vi "DB - [Config].[Messages].vi"(0 "connection reference":T2, 1 "DB Connection":T3={"Open"=TRUE, "Close"=TRUE}, 2 "INSERT TO [SRTRS].[Execute].[MessageLog]":bool, 3 "Application (Default SRTRS)":string="SRTRS", 5 "INSERT TO [AMS].[Execute].[MessageLog]":bool, 7 "Cluster (When DB Not Available)":T1, 9 "<.?...> + Pre-Description<PrePost>Post-Description":string, 11 "error in (no error)":errorcluster) -> (4 "connection reference":T2, 6 "OK Out":bool caption="OK1", 8 "<NoD>":bool, 12 "[Remarks] Pre+Description+Post (Unicode)":string, 13 "Message Code <. ....> FOUND":bool, 14 "[ShortDescription] (Unicode)":string, 15 "SUMMARY":errorcluster)   [LabVIEW 2013]
uses:
  <vilib>/addons/database/Connection.llb/Conn ObjectReference.ctl
  Controls/DB - OpenClose.ctl
  Controls/DB - [SRTRS].[Execute].[MessageLog] ColNames.ctl
  Controls/DB - [AMS].[Execute].[Message] ColNames.ctl
  Controls/Global SRTRS.vi
  <vilib>/addons/database/Connection.llb/DB Tools Open Connec (String).vi
  Controls/Global CMS.vi
  Controls/Global AMS.vi
  <vilib>/addons/database/Connection.llb/Conn Execute.vi
  <vilib>/addons/database/Recordset.llb/Rec Destroy - Connection.vi
  <vilib>/addons/database/NI_Database_API.lvlib
panel:
  out "Config.SG,UG,UGR,Users":string[][](array[string])
  out "Config.SG,UG,UGR,Users":errorcluster
  out "GetNewMessageLogNo":errorcluster
  out "AMS.Execute.Message":errorcluster
  out "[SRTRS].[Execute].[MessageLogNo]":string
  out "AMS.Execute.Message":string="AMS.Execute.MessageLog"
  out "SQL Statement":string[](array[string])
  out "<NoML>":bool
  out "<.....>+ Pre+Description+Post (Unicode)":string
  out "[ShortDescription]":string
  out "[SeverityLevel]":string
  out "Execute.MessageLog":errorcluster
  out "Config.Messages":errorcluster
  out "[MessageId]":string
  out "[MessageType]":string
  out "DB Close Error":errorcluster
  out "Config.Messages":string[](array[string])
  out "DB.Execute.MessageLog":string="SRTRS.Execute.MessageLog"
  out "DB.Config.Messages":string="SRTRS.Config.Messages"
  out "Connection Information":T4={"Connection "="SQL Server 32bit HPEnvy", "Username"="admin", "Password"="admin123"}
  # "<E 602> Hold Temperature Exceeded Variant Allowed!"
  # "Test Codes\nComments\nNeed to set \nPlant, Language\nEnable INSERTS when testing"
  # "<I0101>Admin\n<E7105> Operator<PrePost>4070\n<E8107> Database Not Not Available  (en and zh)"
  # "3C45 2032 3033 3EA2 5B37 620D 54F0 79"
  # "<E7203>ÿþÿþ¢[7b\nTðy Å_{eQ0"
  # "<E 203>¢[7b\nTðy"
  # "[SeverityLevel]                                   [ShortDescription]"
  # "sg.[SeverityGroupId]  ,ug.[UserGroupId] ,ug.[SendSms]  ,ug.[SendEmail]   ,ugr.[UserId]      ,u.[MobileNo]          ,u.[Email]"
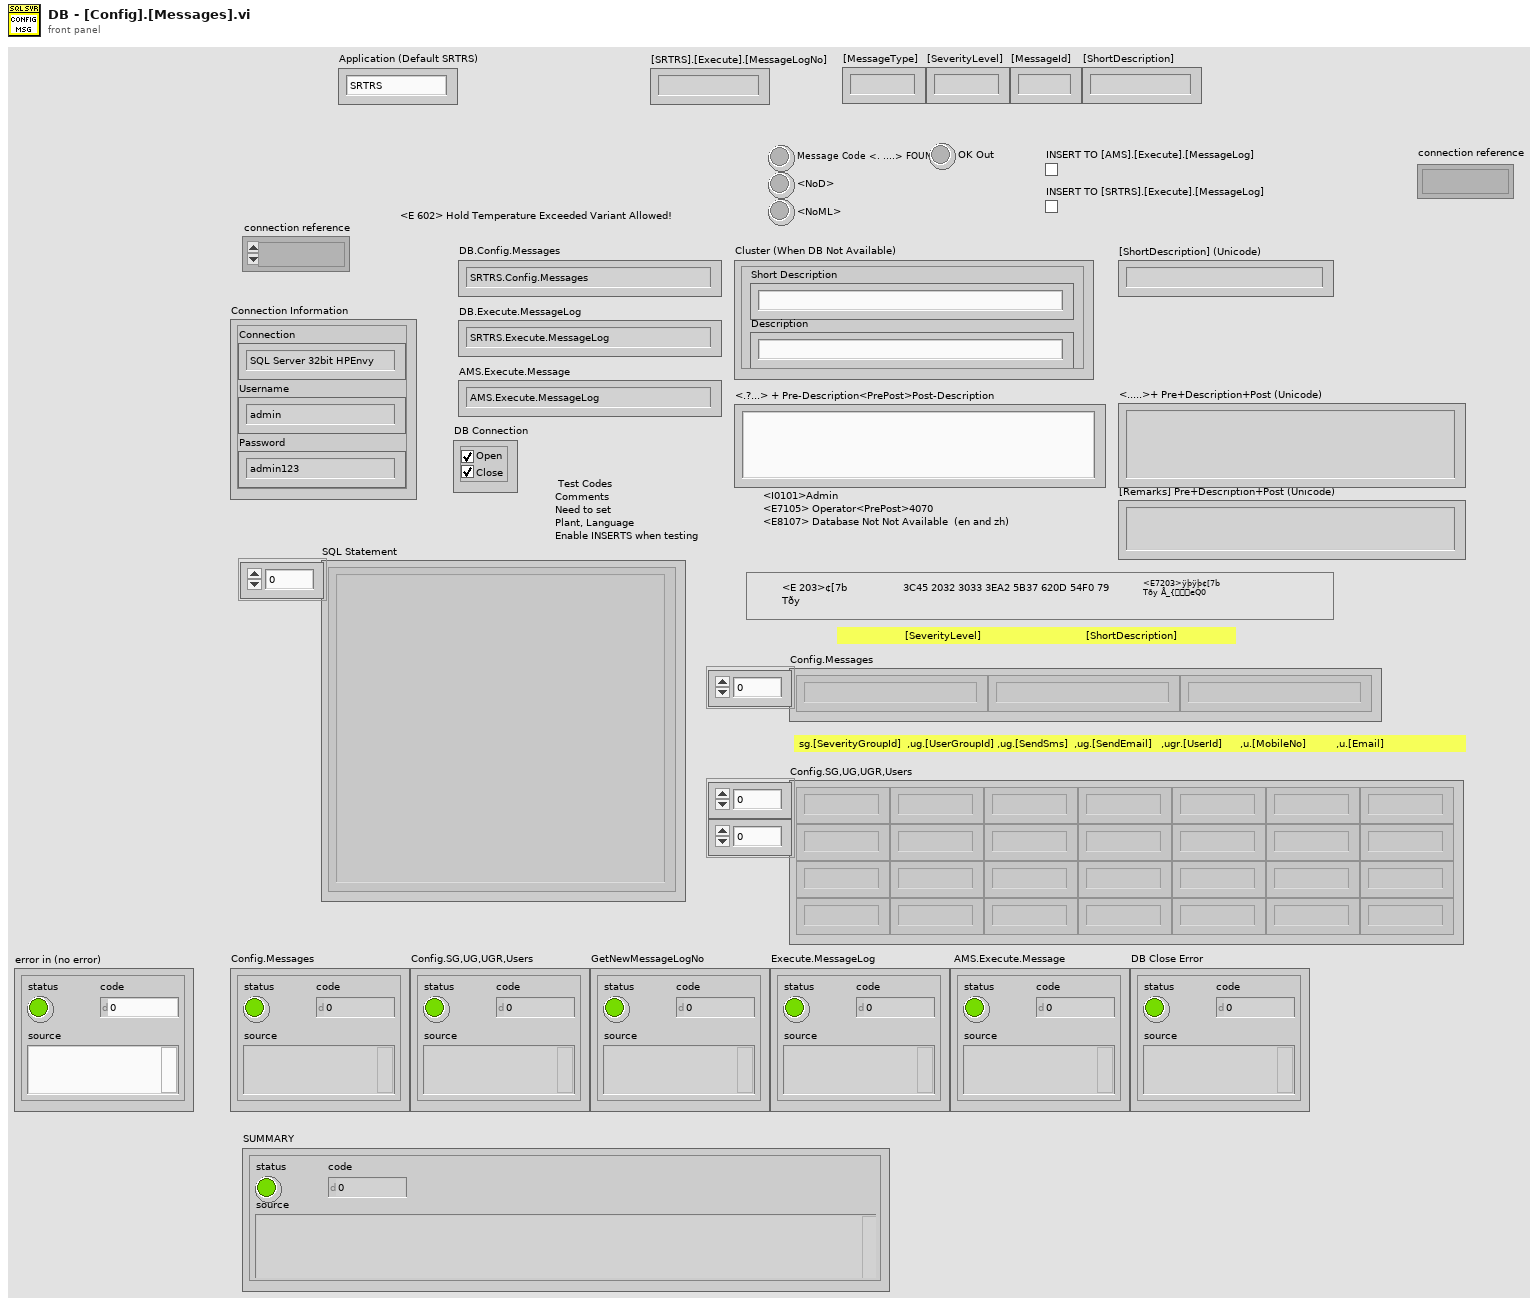
[diagram p1: front panel]
types:
  T1 = cluster{"Short Description":string, "Description":string}
  T2 = typedef "NI_Database_API.lvlib/Conn ObjectReference.ctl" = refnum<k1>
  T3 = typedef "DB - OpenClose.ctl" = cluster{"Open":bool, "Close":bool}
  T4 = cluster{"Connection ":string, "Username":string, "Password":string}
  T5 = typedef "Enum - InteractiveMode-SubVIMode.ctl" = enum16{"Interactive", "subVI Mode"}
  T6 = typedef "DB - Logon Extra Info.ctl" = cluster{"Plant Name":string, "UserName":string, "Hostname [ClientName]":string, "IsUnicode":bool}
  T7 = typedef "Connection Information Cluster.ctl" = cluster{"Connection ":string, "Username":string, "Password":string}
  T8 = typedef "DB - [AMS].[Execute].[Message] ColNames.ctl" = enum16{"[MessageNo]", "[LanguageId]", "[SoftwareSolutionId]", "[SoftwareSolutionName]", "[PlantId]", "[SystemId]", "[StationId]", "[MessageLogNo]", "[ReceivedOn]", "[MessageCode]", "[ShortDescription]", "[Message]", "[SmsMessage]", "[SuppMessage1]", "[SuppMessage2]", "[SuppMessage3]", "[TransactionNo]", "[TransactionRunNo]", "[MessageInitiator]", "[Remarks]", "[MsgCreatedOn]", "[IsToSendSms]", "[IsToSendEmail]", "[IsToSendCommMedium1]", "[IsToSendCommMedium2]", "[SmsContent]", "[EmailContent]", "[CommMed1Content]", "[CommMed2Content]", "[MobileNos]", "[EmailAddresses]", "[CommMedium1Ids]", "[CommMedium2Ids]", "[LastAttemptedCommMed]", "[LastAttemptedNo]", "[LastAttemptedOn]", "[IsSmsSent]", "[IsEmailSent]", "[IsCommMedium1Sent]", "[IsCommMedium2Sent]", "[OverallSentStatus]", "[StatusUpdatedOn]", "[IsArchived]"}
  T9 = typedef "DB - [SRTRS].[Execute].[MessageLog] ColNames.ctl" = enum16{"[MessageLogNo]", "[MessageType]", "[MessageId]", "[SeverityLevel]", "[PlantId]", "[StationId]", "[UserId]", "[TransactionNo]", "[TransactionRunNo]", "[Message]", "[Remarks]", "[CreatedOn]", "[SendRequired]", "[SentOn]", "[OverallMsgStatus]", "[StatusUpdatedOn]", "[IsArchived]"}
  T10 = typedef "DB - Logon Info.ctl" = cluster{"PlantID":string, "SystemID":string, "UserID":string, "DomainID":string, "LanguageID":string, "StationID":string}
  T11 = typedef "DB - DB.Schema.Table.ctl" = cluster{"DB":string, "Schema":string, "Table":string}
  T12 = typedef "NI_Database_API.lvlib/Rec ObjectReference.ctl" = refnum<k1>
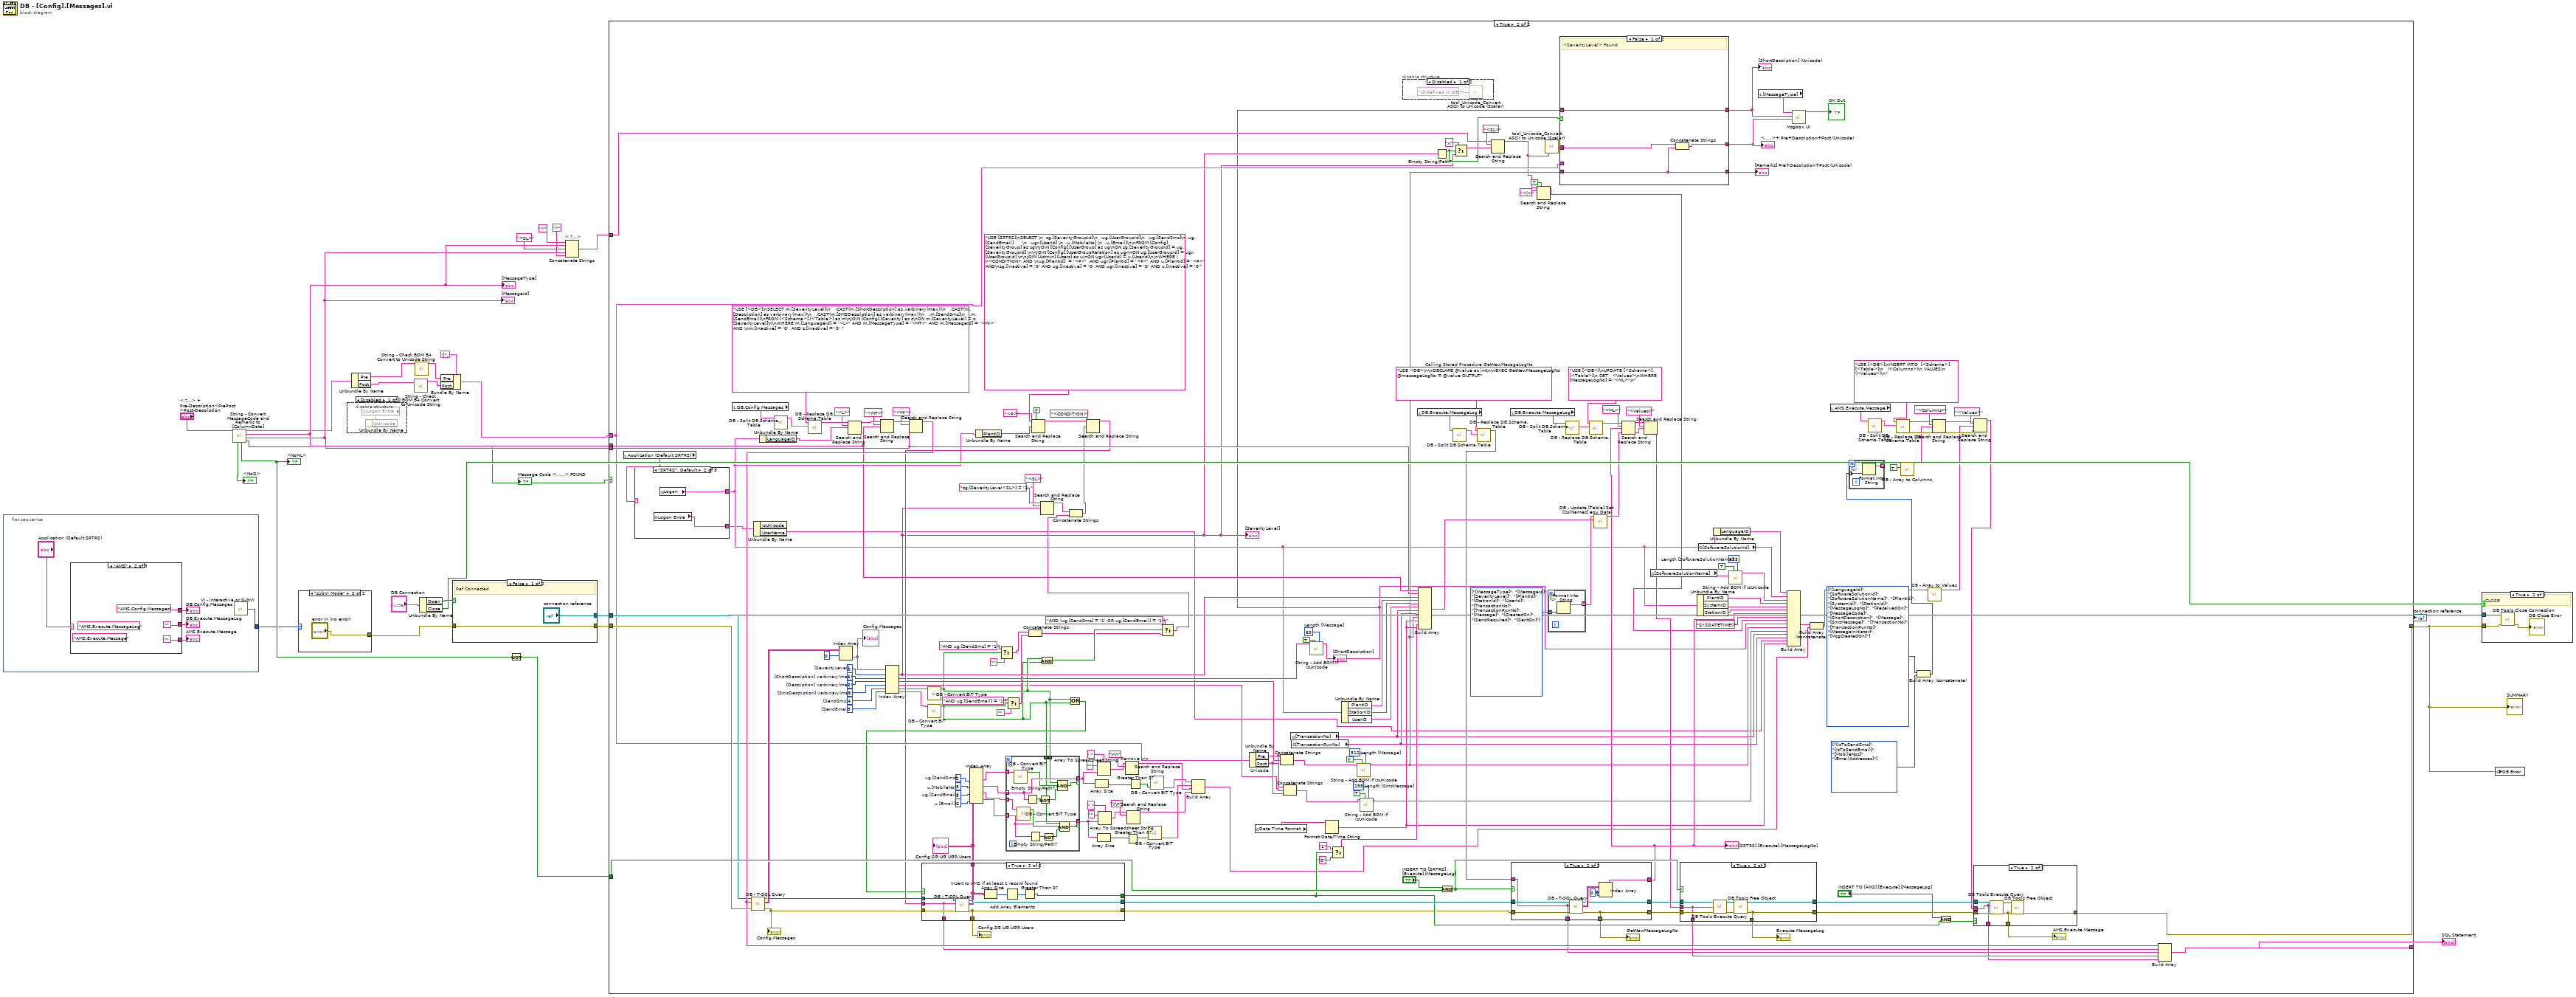
[diagram p0: block diagram]
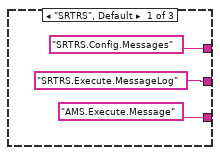
[diagram p2: hidden frame]
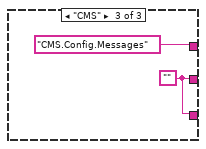
[diagram p3: hidden frame]
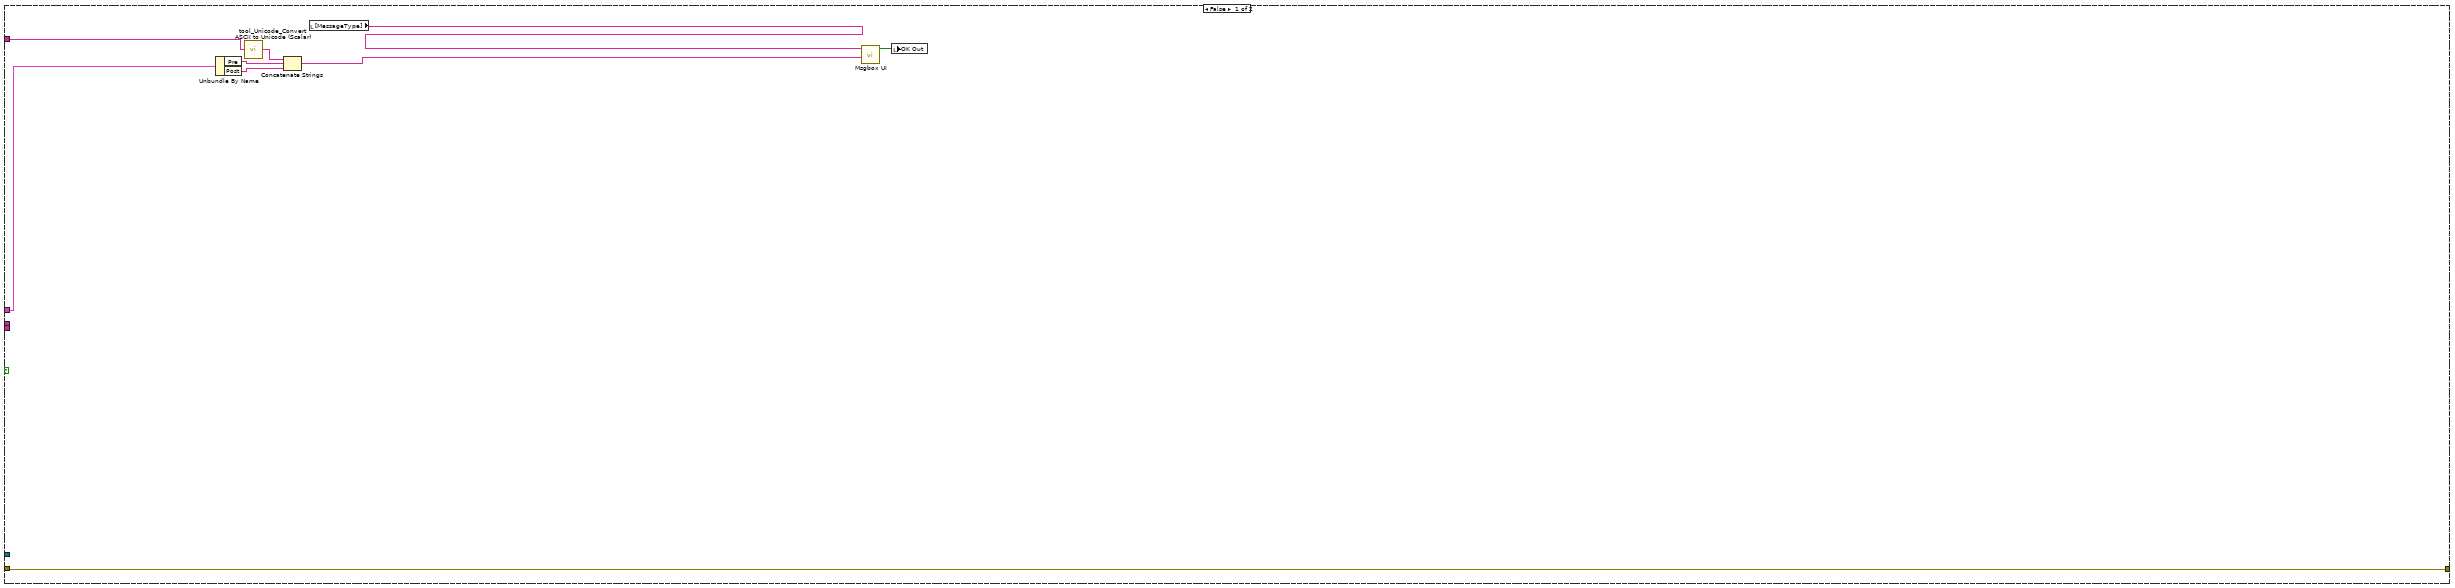
[diagram p5: hidden frame]
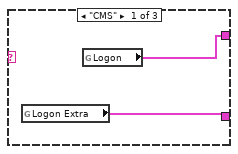
[diagram p6: hidden frame]
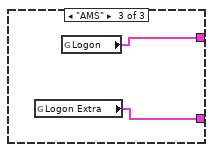
[diagram p7: hidden frame]
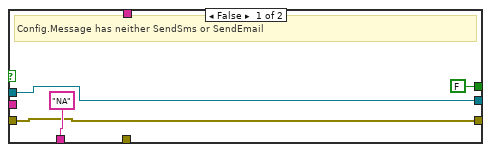
[diagram p8: hidden frame]
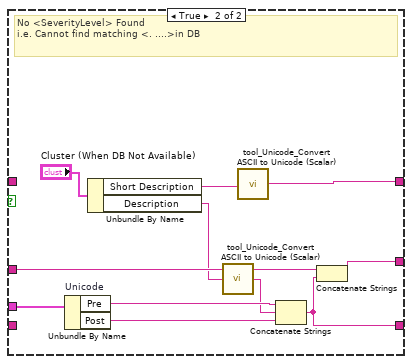
[diagram p9: hidden frame]
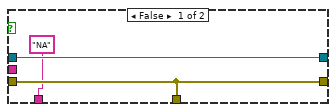
[diagram p11: hidden frame]
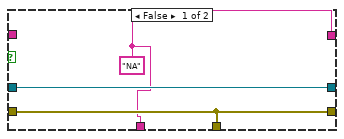
[diagram p12: hidden frame]
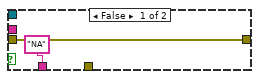
[diagram p13: hidden frame]
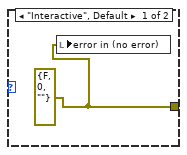
[diagram p15: hidden frame]
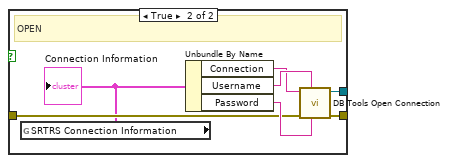
[diagram p16: hidden frame]
diagram:
  n1 = flat-sequence {
    tunnel: [w28] -> w1
    frame #0 {
      n2 = case shown="\"AMS\"" "Application (Default SRTRS)" {
        tunnel: ["SRTRS.Config.Messages" ("SRTRS.Config.Messages") "AMS.Config.Messages" ("SRTRS.Config.Messages") "CMS.Config.Messages" ("SRTRS.Config.Messages")] -> w31
        tunnel: ["SRTRS.Execute.MessageLog" ("SRTRS.Execute.MessageLog") "" w39] -> w30
        tunnel: ["AMS.Execute.Message" ("AMS.Execute.MessageLog") "" w39] -> w29
        frame "SRTRS", Default {
        }
        frame "AMS" {
          (unwired) "AMS.Execute.Message" ("SRTRS.Config.Messages")
          (unwired) "AMS.Execute.MessageLog" ("SRTRS.Config.Messages")
        }
        frame "CMS" {
          w39 = ""
        }
      }
      "DB.Config.Messages" <- w31
      "DB.Execute.MessageLog" <- w30
      "AMS.Execute.Message" <- w29
      n3 = call "VI - Interactive or SubVI.vi"() -> ("Mode"=w28:T5)  [unwired: 5 in]
    }
  }
  n4 = call "String - Convert MessageCode and Remarks to [ColumnData].vi"("<. ....> + Pre-Description<PrePost>Post-Description"="<.?...> + Pre-Description<PrePost>Post-Description") -> ("Message Code <.....> Found"=w10:bool, "[MessageId]"=w18:string, "[MessageType]"=w19:string, "PrePost Description"=w4:cluster{"Pre":string, "Post":string}, "<NoML>"=w11:bool, "<NoD>"=→"<NoD>":bool)  [unwired: 4 in, 1 out]
  "[MessageType]" <- w19
  "[MessageId]" <- w18
  "Message Code <. ....> FOUND" <- w10
  "<NoML>" <- w11
  n5 = case shown="\"subVI Mode\"" w1 {
    tunnel: [w41 "error in (no error)"] -> w25
    frame "Interactive", Default {
      w41 = errorcluster {"status"=FALSE, "code"=0, "source"=""} ("error in (no error)")
      n6 = local write "error in (no error)"(w41) -> ()
    }
    frame "subVI Mode" {
    }
  }
  n7 = disable-structure shown="Disabled" {
    frame Disabled {
      n8 = global read "Global SRTRS.vi" "Logon Extra"() -> (w43:T6)
      n9 = Unbundle By Name(w43) -> ()  [unwired: 1 out]
    }
    frame Enabled {
    }
  }
  n10 = Unbundle By Name ("Depends on IsUnicode")(w4) -> ("Pre"=w7:string, "Post"=w8:string)
  n11 = call "String - Check BOM B4 Convert to Unicode String.vi"("Check 0xFFEE"=w8) -> ("Convert ASCII to Unicode"=w5:string)  [unwired: 10 in]
  n12 = call "String - Check BOM B4 Convert to Unicode String.vi"("Check 0xFFEE"=w7) -> ("Convert ASCII to Unicode"=w6:string)  [unwired: 10 in]
  n13 = Unbundle By Name("DB Connection") -> ("Open"=w26:bool, "Close"=w23:bool)
  n14 = Bundle By Name(cluster=cluster{"Pre":string, "Post":string} {"Pre"="", "Post"=""} ("input cluster"), "Pre"=w6, "Post"=w5) -> (w2:cluster{"Pre":string, "Post":string})
  n15 = case shown="False" w26 {
    tunnel: ["connection reference" w49] -> w12
    tunnel: w25 -> [w44 w48]
    tunnel: [w44 w47] -> w24
    frame False {
      # "Ref Connected"
    }
    frame True {
      # "OPEN"
      n16 = global read "Global SRTRS.vi" "SRTRS Connection Information"() -> (w46:T7)
      "Connection Information" <- w46
      n17 = Unbundle By Name(w46) -> ("Connection"=w51:string, "Username"=w52:string, "Password"=w50:string)
      n18 = call-poly <vilib>:"DB Tools Open Connection.vi"("password"=w50, "userID"=w52, "error in (no error)"=w48, "connection information"=w51) -> ("error out"=w47:errorcluster, "connection reference"=w49:T2)  [unwired: 4 in]
    }
  }
  "connection reference" <- w12
  n19 = Not(x=w11) -> (.not. x?=w15:bool)
  n20 = Concatenate Strings "<.?...>"("<" ("string"), w19, "<SL>" ("search string"), w18, ">" ("string")) -> (w9:string)
  n21 = case shown="True" w10 {
    tunnel: w24 -> [w61 w255]
    tunnel: [w61 w215] -> w21
    tunnel: w19 -> [_ w204]
    tunnel: w18 -> [_ w203]
    tunnel: w15 -> [_ w244]
    tunnel: [_ w243] -> w13
    tunnel: w12 -> [_ w242]
    tunnel: w2 -> [w59 w178]
    tunnel: w9 -> [w55 w185]
    frame False {
      n22 = Unbundle By Name(w59) -> ("Pre"=w58:string, "Post"=w57:string)
      n23 = call "tool_Unicode_Convert ASCII to Unicode (Scalar).vi"("ASCII"=w55) -> ("Unicode"=w54:string)  [unwired: 4 in]
      n24 = Concatenate Strings(w54, w58, w57) -> (w53:string)
      n25 = local read "[MessageType]"() -> (w60:string)
      n26 = call "Msgbox UI.vi"("<xxxxxx> + Pre+Description+Post (Unicode)"=w53, "[MessageType]"=w60) -> ("OK Out"=w56:bool)  [unwired: 7 in, 2 out]
      n27 = local write "OK Out"(w56) -> ()
    }
    frame True {
      w85 = 60  # Length [Message]
      w91 = 255  # Length [SoftwareSolutionName]
      w111 = 5  # [SendEmail
      w112 = 4  # [SendSms]
      w135 = 3  # ug.[SendEmail]
      w139 = 2  # ug.[SendSms]
      w147 = T8[] [enum."[IsToSendSms]", enum."[IsToSendEmail]", enum."[MobileNos]", enum."[EmailAddresses]"] items=["[MessageNo]", "[LanguageId]", "[SoftwareSolutionId]", "[SoftwareSolutionName]", "[PlantId]", "[SystemId]", "[StationId]", "[MessageLogNo]", "[ReceivedOn]", "[MessageCode]", "[ShortDescription]", "[Message]", "[SmsMessage]", "[SuppMessage1]", "[SuppMessage2]", "[SuppMessage3]", "[TransactionNo]", "[TransactionRunNo]", "[MessageInitiator]", "[Remarks]", "[MsgCreatedOn]", "[IsToSendSms]", "[IsToSendEmail]", "[IsToSendCommMedium1]", "[IsToSendCommMedium2]", "[SmsContent]", "[EmailContent]", "[CommMed1Content]", "[CommMed2Content]", "[MobileNos]", "[EmailAddresses]", "[CommMedium1Ids]", "[CommMedium2Ids]", "[LastAttemptedCommMed]", "[LastAttemptedNo]", "[LastAttemptedOn]", "[IsSmsSent]", "[IsEmailSent]", "[IsCommMedium1Sent]", "[IsCommMedium2Sent]", "[OverallSentStatus]", "[StatusUpdatedOn]", "[IsArchived]"]
      w87 = 255  # Length [SmsMessage]
      w149 = 3  # [SmsDescription] varbinary(max)
      w134 = 6  # u.[Email]
      w137 = 5  # u.[MobileNo]
      w192 = 2  # [Description] varbinary(max)
      w88 = 512  # Length [Message]
      w145 = T8[] [enum."[LanguageId]", enum."[SoftwareSolutionId]", enum."[SoftwareSolutionName]", enum."[PlantId]", enum."[SystemId]", enum."[StationId]", enum."[MessageLogNo]", enum."[ReceivedOn]", enum."[MessageCode]", enum."[ShortDescription]", enum."[Message]", enum."[SmsMessage]", enum."[TransactionNo]", enum."[TransactionRunNo]", enum."[MessageInitiator]", enum."[MsgCreatedOn]"] items=["[MessageNo]", "[LanguageId]", "[SoftwareSolutionId]", "[SoftwareSolutionName]", "[PlantId]", "[SystemId]", "[StationId]", "[MessageLogNo]", "[ReceivedOn]", "[MessageCode]", "[ShortDescription]", "[Message]", "[SmsMessage]", "[SuppMessage1]", "[SuppMessage2]", "[SuppMessage3]", "[TransactionNo]", "[TransactionRunNo]", "[MessageInitiator]", "[Remarks]", "[MsgCreatedOn]", "[IsToSendSms]", "[IsToSendEmail]", "[IsToSendCommMedium1]", "[IsToSendCommMedium2]", "[SmsContent]", "[EmailContent]", "[CommMed1Content]", "[CommMed2Content]", "[MobileNos]", "[EmailAddresses]", "[CommMedium1Ids]", "[CommMedium2Ids]", "[LastAttemptedCommMed]", "[LastAttemptedNo]", "[LastAttemptedOn]", "[IsSmsSent]", "[IsEmailSent]", "[IsCommMedium1Sent]", "[IsCommMedium2Sent]", "[OverallSentStatus]", "[StatusUpdatedOn]", "[IsArchived]"]
      w225 = "USE <DB>\n\nDECLARE @value as int\n\nEXEC GetNewMessageLogNo  @messageLogNo = @value OUTPUT"  # Calling Stored Procedure GetNewMesageLogNo
      w229 = T9[] [enum."[MessageType]", enum."[MessageId]", enum."[SeverityLevel]", enum."[PlantId]", enum."[StationId]", enum."[UserId]", enum."[TransactionNo]", enum."[TransactionRunNo]", enum."[Message]", enum."[CreatedOn]", enum."[SendRequired]", enum."[SentOn]"] items=["[MessageLogNo]", "[MessageType]", "[MessageId]", "[SeverityLevel]", "[PlantId]", "[StationId]", "[UserId]", "[TransactionNo]", "[TransactionRunNo]", "[Message]", "[Remarks]", "[CreatedOn]", "[SendRequired]", "[SentOn]", "[OverallMsgStatus]", "[StatusUpdatedOn]", "[IsArchived]"]
      w235 = 1  # [ShortDescription] varbinary(max)
      w239 = 0  # [SeverityLevel]
      n28 = local read "Application (Default SRTRS)"() -> (w80:string)
      n29 = case shown="\"SRTRS\", Default" w80 {
        tunnel: [w257 w259 w261] -> w79
        tunnel: [w256 w258 w260] -> w72
        frame "CMS" {
          n30 = global read "Global CMS.vi" "Logon Extra"() -> (w256:T6)
          n31 = global read "Global CMS.vi" "Logon"() -> (w257:T10)
        }
        frame "SRTRS", Default {
          n32 = global read "Global SRTRS.vi" "Logon Extra"() -> (w258:T6)
          n33 = global read "Global SRTRS.vi" "Logon"() -> (w259:T10)
        }
        frame "AMS" {
          n34 = global read "Global AMS.vi" "Logon Extra"() -> (w260:T6)
          n35 = global read "Global AMS.vi" "Logon"() -> (w261:T10)
        }
      }
      n36 = local read "DB.Config.Messages"() -> (w177:string)
      n37 = Unbundle By Name(w72) -> ("UserName"=w67:string)  [unwired: 1 out]
      n38 = Unbundle By Name(w79) -> ("LanguageID"=w233:string)
      n39 = call "DB - Split DB.Schema.Table.vi"("DB.Schema.Table"=w177) -> ("DB.Schema.Table"=w254:T11)  [unwired: 10 in]
      n40 = call "DB - Replace DB.Schema.Table.vi"("DB.Schema.Table"=w254, "string in"="USE [<DB>]\nSELECT m.[SeverityLevel]\n   ,CAST(m.[ShortDescription] as varbinary(max))\n   ,CAST(m.[Description] as varbinary(max))\n   ,CAST(m.[SMSDescription] as varbinary(max))\n   ,m.[SendSms]\n   ,m.[SendEmail]\nFROM [<Schema>].[<Table>] as m\nJOIN [Config].[Severity] as c\nON m.[SeverityLevel] = c.[SeverityLevel]\n\nWHERE m.[LanguageId] = '<L>' AND m.[MessageType] = '<MT>' AND m.[MessageId] = '<MI>' AND \nm.[Inactive] = '0'  AND c.[Inactive] = '0' ") -> ("string out"=w252:string)  [unwired: 8 in, 1 out]
      n41 = Search and Replace String(input string=w252, search string="<L>", replace string=w233) -> (result string=w250:string)  [unwired: 5 in, 3 out]
      n42 = Search and Replace String(input string=w250, search string="<MT>", replace string=w204) -> (result string=w248:string)  [unwired: 5 in, 3 out]
      n43 = Search and Replace String(input string=w248, search string="<MI>", replace string=w203) -> (result string=w247:string)  [unwired: 5 in, 3 out]
      n44 = call "DB - T-SQL Query.vi"("error in (no error)"=w255, "T-SQL"=w247, "connection reference"=w242) -> ("error out"=w170:errorcluster, "2D data"=w234:string[][], "connection reference"=w171:T2)  [unwired: 6 in]
      "Config.Messages" <- w170
      n45 = Index Array(array=w234, index (row)=0) -> (element=w240:string[])  [unwired: 1 in]
      "Config.Messages" <- w240
      n46 = Index Array(array=w240, index #1=w239, index #2=w235, index #3=w192, index #4=w149, index #5=w112, index #6=w111) -> (element #1=w113:string, element #2=w84:string, element #3=w191:string, element #4=w63:string, element #5=w110:string, element #6=w109:string)
      "[SeverityLevel]" <- w113
      n47 = call "DB - Convert BIT Type.vi"("BIT Type (eg Inactive)"=w110) -> ("Boolean"=w74:bool)  [unwired: 2 in, 2 out]
      n48 = call "DB - Convert BIT Type.vi"("BIT Type (eg Inactive)"=w109) -> ("Boolean"=w73:bool)  [unwired: 2 in, 2 out]
      n49 = Unbundle By Name(w79) -> ("PlantID"=w172:string)
      n50 = Select(t="AND ug.[SendSms] = '1'" ("string (\"\")"), s=w74, f="") -> (s? t:f=w103:string)
      n51 = Select(t="AND ug.[SendEmail] = '1'" ("string (\"\")"), s=w73, f="") -> (s? t:f=w102:string)
      n52 = Concatenate Strings(w103, w102) -> (w76:string)
      n53 = Search and Replace String(replace all?=TRUE ("replace all? (F)"), input string="USE [SRTRS]\nSELECT \n  sg.[SeverityGroupId]\n  ,ug.[UserGroupId]\n  ,ug.[SendSms]\n ,ug.[SendEmail]      \n  ,ugr.[UserId] \n  ,u.[MobileNo] \n  ,u.[Email]\n\nFROM [Config].[SeverityGroup] as sg\nJOIN [Config].[UserGroup] as ug\nON sg.[SeverityGroupId] = ug.[SeverityGroupId] \n\nJOIN [Config].[UserGroupRelation] as ugr\nON ug.[UserGroupId] = ugr.[UserGroupId] \n\nJOIN [Admin].[Users] as u\nON ugr.[UserId] = u.[UserId]\n\nWHERE \n<CONDITION> AND \nug.[PlantId]  = '<P>'  AND ugr.[PlantId] = '<P>' AND u.[PlantId] = '<P>' AND\nsg.[Inactive] = '0' AND ug.[Inactive] = '0' AND ugr.[Inactive] = '0' AND u.[Inactive] = '0'", search string="<P>", replace string=w172) -> (result string=w141:string)  [unwired: 4 in, 3 out]
      n54 = Search and Replace String(input string="sg.[SeverityLevel<SL>] = '1' " ("search string"), search string="<SL>" ("replace string (\"\")"), replace string=w113) -> (result string=w104:string)  [unwired: 5 in, 3 out]
      n55 = And(x=w74, y=w73) -> (x .and. y?=w78:bool)
      n56 = Or(x=w74, y=w73) -> (x .or. y?=w98:bool)
      n57 = Select(t="AND (ug.[SendSms] = '1' OR ug.[SendEmail] = '1') " ("string (\"\")"), s=w78, f=w76) -> (s? t:f=w75:string)
      n58 = Concatenate Strings(w104, w75) -> (w101:string)
      n59 = Search and Replace String(input string=w141, search string="<CONDITION>", replace string=w101) -> (result string=w120:string)  [unwired: 5 in, 3 out]
      n60 = case shown="True" w98 {
        tunnel: w171 -> [w262 w274]
        tunnel: w170 -> [w264 w273]
        tunnel: [_ w266] -> w169
        tunnel: [w262 w272] -> w168
        tunnel: [FALSE w269] -> w167
        tunnel: [_ w268] -> w163
        tunnel: w120 -> [_ w267]
        tunnel: ["NA" ("result string") w267] -> w100
        tunnel: [w264 w266] -> w99
        frame False {
          # "Config.Message has neither SendSms or SendEmail"
        }
        frame True {
          n61 = call "DB - T-SQL Query.vi"("error in (no error)"=w273, "T-SQL"=w267, "connection reference"=w274) -> ("error out"=w266:errorcluster, "2D data"=w268:string[][], "connection reference"=w272:T2)  [unwired: 6 in]
          n62 = Array Size "Insert to AMS if at least 1 record found"(array=w268) -> (size(s)=w271:i32[])
          n63 = Add Array Elements(numeric array=w271) -> (sum=w270:i32)
          n64 = Greater Than 0?(x=w270) -> (x > 0?=w269:bool)
        }
      }
      "Config.SG,UG,UGR,Users" <- w169
      "Config.SG,UG,UGR,Users" <- w163
      n65 = Index Array(array=w163, index (col) #1=w139, index (col) #2=w137, index (col) #3=w135, index (col) #4=w134) -> (element #1=w138:string[], element #2=w136:string[], element #3=w133:string[], element #4=w132:string[])  [unwired: 4 in]
      n66 = for {
        tunnel: w138 -> [w288] mode=indexing
        tunnel: w136 -> [w287] mode=indexing
        tunnel: [w287] -> w131 mode=indexing if=w283
        tunnel: w133 -> [w282] mode=indexing
        tunnel: w132 -> [w278] mode=indexing
        tunnel: [w278] -> w130 mode=indexing if=w277
        tunnel: w74 -> [w276]
        tunnel: w73 -> [w275]
        n67 = call "DB - Convert BIT Type.vi"("BIT Type (eg Inactive)"=w288) -> ("Boolean"=w285:bool)  [unwired: 2 in, 2 out]
        n68 = call "DB - Convert BIT Type.vi"("BIT Type (eg Inactive)"=w282) -> ("Boolean"=w280:bool)  [unwired: 2 in, 2 out]
        n69 = Empty String/Path?(string/path=w287) -> (empty?=w286:bool)
        n70 = Empty String/Path?(string/path=w278) -> (empty?=w281:bool)
        n71 = Not(x=w286) -> (.not. x?=w284:bool)
        n72 = Not(x=w281) -> (.not. x?=w279:bool)
        n73 = Compound Arithmetic op=AND(w276, w285, w284) -> (w283:bool)
        n74 = Compound Arithmetic op=AND(w275, w280, w279) -> (w277:bool)
      }
      n75 = Array Size(array=w131) -> (size(s)=w129:i32)
      n76 = Array To Spreadsheet String(delimiter (Tab)=",", array=w131, 3:"" ("format string")) -> (spreadsheet string=w156:string)
      n77 = Array Size(array=w130) -> (size(s)=w128:i32)
      n78 = Array To Spreadsheet String(delimiter (Tab)=",", array=w130, 3:"" ("format string")) -> (spreadsheet string=w157:string)
      n79 = Search and Replace String "Remove \\r\\n"(input string=w156, search string="\r\n") -> (result string=w123:string)  [unwired: 6 in, 3 out]
      n80 = Greater Than 0?(x=w128) -> (x > 0?=w126:bool)
      n81 = Search and Replace String(input string=w157, search string="\r\n") -> (result string=w122:string)  [unwired: 6 in, 3 out]
      n82 = Greater Than 0?(x=w129) -> (x > 0?=w127:bool)
      n83 = call "DB - Convert BIT Type.vi"("Boolean"=w126) -> ("BIT (eg Inactive)"=w124:string)  [unwired: 2 in, 2 out]
      n84 = call "DB - Convert BIT Type.vi"("Boolean"=w127) -> ("BIT (eg Inactive)"=w125:string)  [unwired: 2 in, 2 out]
      n85 = Build Array(w125, w124, w123, w122) -> (w121:string[])
      n86 = Unbundle By Name "Unicode"(w178) -> ("Pre"=w65:string, "Post"=w64:string)
      n87 = global read "Global SRTRS.vi" "Date Time Format"() -> (w237:string)
      n88 = Concatenate Strings(w65, w191, w64) -> (w90:string)
      n89 = Concatenate Strings(w65, w63, w64) -> (w62:string)
      n90 = global read "Global SRTRS.vi" "[TransactionNo]"() -> (w197:string)
      n91 = global read "Global SRTRS.vi" "[TransactionRunNo]"() -> (w196:string)
      n92 = call "String - Add BOM if IsUnicode.vi"("target length (65535)"=w85, "Input is Unicode (varbinary)?"=TRUE ("IsUnicode?"), "String IN"=w84) -> ("BOM Added"=w83:string)  [unwired: 8 in]
      "[ShortDescription]" <- w83
      n93 = Format Date/Time String(time format string (%c)=w237) -> (date/time string=w148:string)  [unwired: 2 in]
      n94 = Select(t="1", s=w167, f="0") -> (s? t:f=w164:string)
      n95 = Unbundle By Name(w79) -> ("PlantID"=w202:string, "StationID"=w198:string, "UserID"=w66:string)
      n96 = call "String - Add BOM if IsUnicode.vi"("target length (65535)"=w88, "Input is Unicode (varbinary)?"=TRUE, "String IN"=w90) -> ("BOM Added"=w89:string)  [unwired: 8 in]
      n97 = call "String - Add BOM if IsUnicode.vi"("target length (65535)"=w87, "Input is Unicode (varbinary)?"=TRUE, "String IN"=w62) -> ("BOM Added"=w86:string)  [unwired: 8 in]
      n98 = disable-structure shown="Disabled" {
        frame Disabled {
          n99 = call "tool_Unicode_Convert ASCII to Unicode (Scalar).vi"("ASCII"="Undefined in DB.") -> ()  [unwired: 4 in, 1 out]
        }
        frame Enabled {
        }
      }
      n100 = local read "DB.Execute.MessageLog"() -> (w176:string)
      n101 = Build Array(w204, w203, w113, w202, w198, w66, w197, w196, w89, w148, w164, w148) -> (w230:string[])
      n102 = Empty String/Path?(string/path=w113) -> (empty?=w181:bool)
      n103 = And(x="INSERT TO [SRTRS].[Execute].[MessageLog]", y=w244) -> (x .and. y?=w194:bool)
      n104 = call "DB - Split DB.Schema.Table.vi"("DB.Schema.Table"=w176) -> ("DB.Schema.Table"=w226:T11)  [unwired: 10 in]
      n105 = Select(t="x", s=w181, f=w113) -> (s? t:f=w188:string)
      n106 = call "DB - Replace DB.Schema.Table.vi"("DB.Schema.Table"=w226, "string in"=w225) -> ("string out"=w224:string)  [unwired: 8 in, 1 out]
      n107 = Search and Replace String(input string=w185, search string="<SL>", replace string=w188) -> (result string=w95:string)  [unwired: 5 in, 3 out]
      n108 = local read "DB.Execute.MessageLog"() -> (w219:string)
      n109 = case shown="True" w194 {
        tunnel: w168 -> [w317 w325]
        tunnel: w99 -> [w316 w324]
        tunnel: w224 -> [_ w318]
        tunnel: [w315 w321] -> w151
        tunnel: [w317 w320] -> w200
        tunnel: [w316 w319] -> w195
        tunnel: [w316 w319] -> w193
        tunnel: [w315 w318] -> w119
        frame False {
          w315 = "NA" ("String")
        }
        frame True {
          w322 = 0
          n110 = call "DB - T-SQL Query.vi"("error in (no error)"=w324, "T-SQL"=w318, "connection reference"=w325) -> ("error out"=w319:errorcluster, "2D data"=w323:string[][], "connection reference"=w320:T2)  [unwired: 6 in]
          n111 = Index Array(array=w323, index (row)=w322, index (col)=w322) -> (element=w321:string)
        }
      }
      "[SRTRS].[Execute].[MessageLogNo]" <- w151
      "GetNewMessageLogNo" <- w195
      n112 = Search and Replace String(replace all?=TRUE ("replace all? (F)"), input string=w95, search string="<|>") -> (result string=w94:string)  [unwired: 5 in, 3 out]
      n113 = call "tool_Unicode_Convert ASCII to Unicode (Scalar).vi"("ASCII"=w95) -> ("Unicode"=w189:string)  [unwired: 4 in]
      n114 = for {
        tunnel: w229 -> [w337] mode=indexing
        tunnel: [w336] -> w228 mode=indexing
        n115 = Format Into String(w337) -> (resulting string=w336:string)  [unwired: 3 in, 1 out]
      }
      n116 = case shown="False" w181 {
        tunnel: w189 -> [w292 w303]
        tunnel: [w291 w298] -> w183
        tunnel: w89 -> [w289 _]
        tunnel: w83 -> [w290 _]
        tunnel: [w290 w299] -> w180
        tunnel: [w289 w293] -> w179
        tunnel: w178 -> [_ w297]
        frame False {
          # "<SeverityLevel> Found"
          n117 = Concatenate Strings(w292, w289) -> (w291:string)
        }
        frame True {
          # "No <SeverityLevel> Found\ni.e. Cannot find matching <. ....>in DB"
          n118 = Unbundle By Name "Unicode"(w297) -> ("Pre"=w296:string, "Post"=w294:string)
          n119 = Unbundle By Name("Cluster (When DB Not Available)") -> ("Short Description"=w301:string, "Description"=w300:string)
          n120 = call "tool_Unicode_Convert ASCII to Unicode (Scalar).vi"("ASCII"=w300) -> ("Unicode"=w295:string)  [unwired: 4 in]
          n121 = call "tool_Unicode_Convert ASCII to Unicode (Scalar).vi"("ASCII"=w301) -> ("Unicode"=w299:string)  [unwired: 4 in]
          n122 = Concatenate Strings(w296, w295, w294) -> (w293:string)
          n123 = Concatenate Strings(w303, w293) -> (w298:string)
        }
      }
      "<.....>+ Pre+Description+Post (Unicode)" <- w183
      "[ShortDescription] (Unicode)" <- w180
      "[Remarks] Pre+Description+Post (Unicode)" <- w179
      n124 = call "DB - Split DB.Schema.Table.vi"("DB.Schema.Table"=w219) -> ("DB.Schema.Table"=w245:T11)  [unwired: 10 in]
      n125 = call "DB - Replace DB.Schema.Table.vi"("DB.Schema.Table"=w245, "string in"="USE [<DB>]\nUPDATE [<Schema>].[<Table>]\n SET   <Values>\nWHERE [MessageLogNo] = '<ML>'\n") -> ("string out"=w223:string)  [unwired: 8 in, 1 out]
      n126 = call "DB - Update [Table] Set [ColNames] equ Data.vi"("<Data> (0xFFFE autodetect)"=w230, "[ColumnNames]"=w228) -> ("<Values>"=w227:string)  [unwired: 9 in]
      n127 = Search and Replace String(input string=w223, search string="<ML>", replace string=w151) -> (result string=w221:string)  [unwired: 5 in, 3 out]
      n128 = Search and Replace String(input string=w221, search string="<Values>", replace string=w227) -> (result string=w150:string)  [unwired: 5 in, 3 out]
      n129 = global read "Global SRTRS.vi" "[SoftwareSolutionName]"() -> (w93:string)
      n130 = case shown="True" w194 {
        tunnel: [w306 w309] -> w236
        tunnel: w150 -> [_ w308]
        tunnel: [w306 w309] -> w216
        tunnel: [w307 w313] -> w213
        tunnel: w200 -> [w307 w312]
        tunnel: w193 -> [w306 w311]
        tunnel: ["NA" ("result string") w308] -> w118
        frame False {
        }
        frame True {
          n131 = call-poly <vilib>:"DB Tools Execute Query.vi"("error in (no error)"=w311, "SQL query"=w308, "connection reference"=w312) -> ("error out"=w314:errorcluster, "recordset reference"=w310:T12)  [unwired: 5 in]
          n132 = call-poly <vilib>:"DB Tools Free Object.vi"("error in (no error)"=w314, "recordset reference"=w310) -> ("error out"=w309:errorcluster, "connection reference"=w313:T2)  [unwired: 8 in]
        }
      }
      "Execute.MessageLog" <- w236
      n133 = Unbundle By Name(w79) -> ("PlantID"=w155:string, "SystemID"=w154:string, "StationID"=w153:string)
      n134 = global read "Global SRTRS.vi" "[SoftwareSolutionId]"() -> (w201:string)
      n135 = Unbundle By Name(w79) -> ("LanguageID"=w82:string)
      n136 = call "String - Add BOM if IsUnicode.vi"("target length (65535)"=w91, "Input is Unicode (varbinary)?"=TRUE, "String IN"=w93) -> ("BOM Added"=w92:string)  [unwired: 8 in]
      n137 = local read "[MessageType]"() -> (w184:string)
      n138 = Build Array(w82, w201, w92, w155, w154, w153, w151, "SYSDATETIME()" ("[ReceivedOn]"), w94, w83, w89, w86, w197, w196, w67, w148) -> (w144:string[])
      n139 = call "Msgbox UI.vi"("<xxxxxx> + Pre+Description+Post (Unicode)"=w183, "[ShortDescription] (Unicode)"=w180, "[MessageType]"=w184) -> ("OK Out"=→"OK Out":bool)  [unwired: 6 in, 2 out]
      n140 = Build Array (concatenate)(w144, w121) -> (w143:string[])
      n141 = local read "AMS.Execute.Message"() -> (w175:string)
      n142 = call "DB - Split DB.Schema.Table.vi"("DB.Schema.Table"=w175) -> ("DB.Schema.Table"=w232:T11)  [unwired: 10 in]
      n143 = call "DB - Replace DB.Schema.Table.vi"("DB.Schema.Table"=w232, "string in"="USE [<DB>]\nINSERT INTO  [<Schema>].[<Table>]\n   (<Columns>)\n VALUES\n  (<Values>)\n") -> ("error out"=w211:errorcluster, "string out"=w208:string)  [unwired: 8 in]
      n144 = Build Array (concatenate)(w145, w147) -> (w146:T8[])
      n145 = for {
        tunnel: w146 -> [w327] mode=indexing
        tunnel: [w326] -> w205 mode=indexing
        n146 = Format Into String(w327) -> (resulting string=w326:string)  [unwired: 3 in, 1 out]
      }
      n147 = call "DB - Array to Columns.vi"("Exclude []"=TRUE, "Array"=w205) -> ("[Columns]"=w206:string)  [unwired: 9 in]
      n148 = call "DB - Array to Values.vi"("Array (0xFFFE autodetect)"=w143) -> ("<Values>"=w210:string)  [unwired: 10 in]
      n149 = Search and Replace String(input string=w208, search string="<Columns>", replace string=w206) -> (result string=w207:string)  [unwired: 5 in, 3 out]
      n150 = And(x="INSERT TO [AMS].[Execute].[MessageLog]", y=w167) -> (x .and. y?=w218:bool)
      n151 = Search and Replace String(input string=w207, search string="<Values>", replace string=w210, error in=w211) -> (result string=w117:string)  [unwired: 4 in, 3 out]
      n152 = case shown="True" w218 {
        tunnel: w216 -> [w329 w334]
        tunnel: [w329 w333] -> w215
        tunnel: [_ w332] -> w214
        tunnel: w213 -> [_ w331]
        tunnel: w117 -> [_ w330]
        tunnel: ["NA" ("result string") w330] -> w116
        frame False {
        }
        frame True {
          n153 = call-poly <vilib>:"DB Tools Execute Query.vi"("error in (no error)"=w334, "SQL query"=w330, "connection reference"=w331) -> ("error out"=w332:errorcluster, "recordset reference"=w335:T12)  [unwired: 5 in]
          n154 = call-poly <vilib>:"DB Tools Free Object.vi"("error in (no error)"=w332, "recordset reference"=w335) -> ("error out"=w333:errorcluster)  [unwired: 8 in, 1 out]
        }
      }
      "AMS.Execute.Message" <- w214
      n155 = Build Array(w247, w100, w119, w118, w116) -> (w243:string[])
    }
  }
  "SUMMARY" <- w21
  "SQL Statement" <- w13
  n156 = case shown="True" w23 {
    tunnel: w12 -> [_ w340]
    tunnel: w21 -> [_ w338]
    frame False {
      # "Ref Connected"
    }
    frame True {
      # "CLOSE"
      n157 = call <vilib>:"DB Tools Close Connection.vi"("error in (no error)"=w338, "connection reference"=w340) -> ("error out"=→"DB Close Error":errorcluster)  [unwired: 5 in]
    }
  }
  n158 = global write "Global SRTRS.vi" "DB Error"(w21) -> ()
